vi "BIO_free_all.vi"(8 "error in (no error)":errorcluster, 11 "BIO in":refnum<class "BIO.lvclass">) -> (0 "error out":errorcluster)   [LabVIEW 2013, in "OpenSSL Socket.lvlib" / "BIO.lvclass"]
uses:
  BIO.lvclass
  SSL-Lib/SSL-Lib.lvclass/SSL-Lib.ctl
  BIO.lvclass/BIO.ctl
  SSL-Lib/Read Crypto Library Path.vi
  Read Handle.vi
  SSL-Lib/SSL-Lib.lvclass
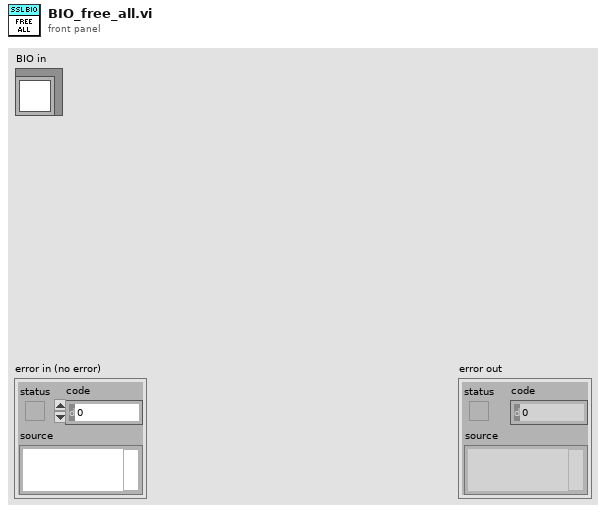
[diagram p1: front panel]
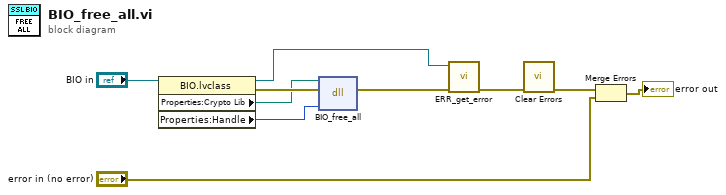
[diagram p0: block diagram]
diagram:
  n1 = property class="BIO.lvclass"(reference="BIO in") -> (reference out=w4:refnum<class "BIO.lvclass">, error out=w9:errorcluster, "Properties:Crypto Lib"=w8:path, "Properties:Handle"=w7:u64)  [unwired: 1 in]
  n2 = dll-call lib="C:/Program Files (x86)/National Instruments/Shared/nissl/NIlibeay32.dll" fn="BIO_free_all"(path in=w8, error in=w9, "BIO"=w7) -> (error out=w5:errorcluster)  [unwired: 3 in, 1 out]
  n3 = call "ERR_get_error.vi"("error in (no error)"=w5, "SSL-Lib in"=w4) -> ("error out"=w3:errorcluster)  [unwired: 8 in, 1 out]
  n4 = call <vilib>:"Clear Errors.vi"("error in (no error)"=w3) -> ("error out"=w1:errorcluster)  [unwired: 6 in]
  n5 = Merge Errors(w1, "error in (no error)") -> (→"error out":errorcluster)
